vi "Create (Element).vi"(8 "error in (no error)":errorcluster, 10 "Element":refnum<class "Config Element.lvclass">, 11 "VolatusConfigElement in":refnum<class "VolatusConfigElement.lvclass">) -> (0 "error out":errorcluster, 3 "VolatusConfigElement out":refnum<class "VolatusConfigElement.lvclass">)   [LabVIEW 2020, in "VolatusConfig.lvlib" / "VolatusConfigElement.lvclass"]
uses:
  VolatusConfigElement.lvclass
  lv-cdm/CDM-Config/Config Element/Config Element.lvclass
  VolatusConfigElement.lvclass/VolatusConfigElement.ctl
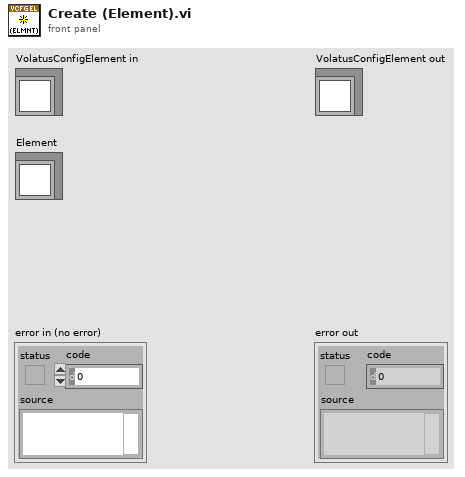
[diagram p1: front panel]
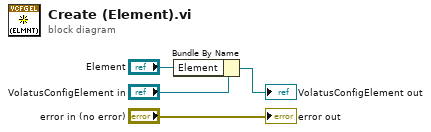
[diagram p0: block diagram]
diagram:
  n1 = Bundle By Name(cluster="VolatusConfigElement in", "Element"="Element") -> (→"VolatusConfigElement out":refnum<class "VolatusConfigElement.lvclass">)
  "error out" <- "error in (no error)"
